vi "Lab Panel V5.40.vi"() -> ()   [LabVIEW 2017] (continued)
                                frame "CHART TEST", Default {
                                }
                                frame "CYCLE TEST" {
                                }
                                frame "T-RISE TEST" {
                                }
                                }
                                n851 = Unbundle(w1495) -> ("DESCRIPTION"=w1494:string)  [unwired: 4 out]
                                n852 = Concatenate Strings(w1490, "\\", w1488, w1486, w1487, w1486) -> (w1497:string)
                                n853 = String To Path(string=w1497) -> (path=w1499:path)
                                n854 = Concatenate Strings(w1497, w1496, w1494, "-", w1493, ".tdms") -> (w1485:string)
                                n855 = Create Folder(path (use dialog)=w1499) -> (error out=w1498:errorcluster)  [unwired: 2 in, 2 out]
                                n856 = global write "Global 1.vi" "LAB03-2 FILE"(w1485) -> ()
                                n857 = call <vilib>:"Clear Errors.vi"("error in (no error)"=w1498) -> ()  [unwired: 5 in, 2 out]
                              }
                              frame #1 {
                                (unwired) FALSE
                                n858 = String To Path(string=w1509) -> (path=w1505:path)
                                n859 = TDMS Open(6:FALSE, 10:T22."create or replace" ("operation (0:open)"), 11:w1505) -> (0:w1504:errorcluster, 3:→"TDMS LAB03-2":refnum<k34>)  [unwired: 4 in]
                              }
                              frame #2 {
                                n860 = local read "SET LAB03-2"() -> (w1515:T5)
                                n861 = local read "TDMS LAB03-2"() -> (w1526:refnum<k34>)
                                n862 = Build Array("Testers Name", "Description", "Set Test Cycles", "T-Rise minutes", "T-Rise Deg C") -> (w1516:string[])
                                n863 = Unbundle(w1515) -> ("NAME"=w1514:string, "DESCRIPTION"=w1513:string, "CYCLES"=w1512:dbl, "T-RISE mins"=w1511:dbl, "T-RISE deg C"=w1510:dbl)
                                n864 = Number To Decimal String(number=w1512) -> (decimal integer string=w1525:string)  [unwired: 1 in]
                                n865 = Number To Decimal String(number=w1511) -> (decimal integer string=w1524:string)  [unwired: 1 in]
                                n866 = Number To Decimal String(number=w1510) -> (decimal integer string=w1523:string)  [unwired: 1 in]
                                n867 = Build Array(w1514, w1513, w1525, w1524, w1523) -> (w1522:string[])
                                n868 = TDMS Set Properties(5:w1522, 7:w1516, 11:w1526) -> ()  [unwired: 3 in, 4 out]
                              }
                              frame #3 {
                                n869 = local read "DISP LAB03-2"() -> (w1531:T4)
                                n870 = Concatenate Strings("LAB03-2  ", w1530) -> (w1532:string)
                                n871 = Two Button Dialog(message=w1532, 1:w1528, 2:w1529) -> (T button?=w1534:bool)
                                n872 = case shown="True" w1534 {
                                tunnel: w1531 -> [w1541 w1542]
                                tunnel: [w1541 w1542] -> w1538
                                tunnel: [w1540 w1543] -> w1537
                                tunnel: [w1539 w1543] -> w1536
                                frame False {
                                n873 = Unbundle(w1541) -> ("CYCLE"=w1540:dbl, "MINS"=w1539:dbl)  [unwired: 1 out]
                                }
                                frame True {
                                w1543 = 0.0
                                }
                                }
                                n874 = Bundle(cluster=w1538, "CYCLE"=w1537, "MINS"=w1536, "STATUS"="RUN") -> (w1527:T4)
                                n875 = local write "DISP LAB03-2"(w1527) -> ()
                              }
                              frame #4 {
                                n876 = local read "TEMP START LAB03-2"() -> (w1546:cluster{"TL":dbl, "TN":dbl})
                                n877 = Bundle(cluster=w1546, "TL"=w1544, "TN"=w1544) -> (w1545:cluster{"TL":dbl, "TN":dbl})
                                n878 = local write "TEMP START LAB03-2"(w1545) -> ()
                              }
                            }
                          }
                        }
                      }
                    }
                  }
                }
              }
              event "RUN LAB04-1": Value Change {
                n879 = event-data() -> ("NewVal"=w1551:bool)  [unwired: 1 in, 5 out]
                n880 = local write "run lab04-1"(w1551) -> ()
                n881 = case shown="True" w1551 {
                  tunnel: w1557 -> [_ w1595]
                  tunnel: w1556 -> [_ w1594]
                  tunnel: w1554 -> [w1559 w1593]
                  tunnel: w1555 -> [_ w1592]
                  tunnel: w1553 -> [_ w1591]
                  tunnel: [w1558 w1590] -> w1552
                  tunnel: w1550 -> [_ w1589]
                  tunnel: w1549 -> [_ w1588]
                  tunnel: w1548 -> [_ w1587]
                  tunnel: w1547 -> [_ w1585]
                  frame False {
                    # "stop test"
                    n882 = stacked-sequence {
                      tunnel: w1559 -> [w1568 _]
                      tunnel: [w1560 _] -> w1558
                      frame #0 {
                        n883 = local read "DISP LAB04-1"() -> (w1567:T4)
                        n884 = Unbundle(w1567) -> ("CYCLE"=w1565:dbl, "MINS"=w1566:dbl)  [unwired: 1 out]
                        n885 = case shown="\"CYCLE TEST\"" w1568 {
                          tunnel: w1566 -> [_ _ w1575]
                          tunnel: w1565 -> [w1573 w1574 _]
                          tunnel: [w1573 w1574 w1575] -> w1564
                          frame "CHART TEST", Default {
                          }
                          frame "CYCLE TEST" {
                          }
                          frame "T-RISE TEST" {
                          }
                        }
                        n886 = local read "TDMS LAB04-1"() -> (w1572:refnum<k34>)
                        n887 = Build Array("STOPPED") -> (w1569:string[])
                        n888 = Build Array(w1564) -> (w1563:dbl[])
                        n889 = TDMS Write(0:w1572, 5:"TEST RESULT", 7:w1569, 9:w1563) -> (4:w1561:refnum<k34>, 15:w1562:errorcluster)  [unwired: 2 in, 2 out]
                        n890 = TDMS Close(8:w1562, 11:w1561) -> (0:w1560:errorcluster)  [unwired: 1 out]
                      }
                      frame #1 {
                        n891 = local read "DISP LAB04-1"() -> (w1579:T4)
                        n892 = stacked-sequence {
                          tunnel: "LAB04-1" -> [w1581 w1583]
                          frame #0 {
                            n893 = call "sub vi - defrag tdms v1.vi"("panel id"=w1581) -> ("error out"=w1580:errorcluster)  [unwired: 10 in]
                            n894 = local write "data file error"(w1580) -> ()
                          }
                          frame #1 {
                            n895 = call "Save data file (stop) v3.vi"("panel id"=w1583) -> ("network file save error"=w1582:errorcluster)  [unwired: 9 in, 1 out]
                            n896 = local write "RESULT LAB04-1"(FALSE) -> ()
                            n897 = local write "data file error"(w1582) -> ()
                          }
                        }
                        n898 = Bundle(cluster=w1579, "STATUS"="STOP") -> (w1577:T4)  [unwired: 2 in]
                        n899 = local write "DISP LAB04-1"(w1577) -> ()
                      }
                    }
                  }
                  frame True {
                    n900 = local read "SIG LAB04-1"() -> (w1586:T2)
                    n901 = stacked-sequence {
                      seq-local: [w1597 _] -> [_ w1601]
                      tunnel: w1595 -> [_ w1611]
                      tunnel: w1594 -> [_ w1610]
                      tunnel: w1593 -> [_ w1609]
                      tunnel: w1592 -> [_ w1608]
                      tunnel: w1591 -> [_ w1607]
                      tunnel: [_ w1606] -> w1590
                      tunnel: w1589 -> [_ w1605]
                      tunnel: w1588 -> [_ w1604]
                      tunnel: w1587 -> [_ w1603]
                      tunnel: w1586 -> [w1596 w1602]
                      tunnel: w1585 -> [_ w1600]
                      frame #0 {
                        n902 = Unbundle(w1596) -> ("AMPS"=w1599:dbl)  [unwired: 4 out]
                        n903 = call "Check For Amps on v1.vi"("ID"="LAB04-1", "amps"=w1599) -> ("amps"=w1597:bool)  [unwired: 9 in]
                      }
                      frame #1 {
                        n904 = case shown="True" w1601 {
                          tunnel: w1611 -> [_ w1624]
                          tunnel: w1610 -> [_ w1623]
                          tunnel: w1609 -> [_ w1622]
                          tunnel: w1608 -> [_ w1621]
                          tunnel: w1607 -> [_ w1620]
                          tunnel: [errorcluster {"status"=FALSE, "code"=0, "source"=""} ("error out") w1619] -> w1606
                          tunnel: w1605 -> [_ w1618]
                          tunnel: w1604 -> [_ w1617]
                          tunnel: w1603 -> [_ w1616]
                          tunnel: w1602 -> [_ w1615]
                          tunnel: w1600 -> [_ w1614]
                          frame False {
                            w1612 = FALSE
                            n905 = local write "RUN LAB04-1"(w1612) -> ()
                            n906 = local write "run lab04-1"(w1612) -> ()
                          }
                          frame True {
                            n907 = stacked-sequence {
                              seq-local: [w1625 _ _ _ _] -> [_ w1649 _ _ _]
                              tunnel: w1624 -> [w1630 _ _ _ _]
                              tunnel: w1623 -> [w1626 _ _ _ _]
                              tunnel: w1622 -> [w1640 _ _ _ _]
                              tunnel: w1621 -> [w1633 _ _ _ _]
                              tunnel: w1620 -> [w1628 _ _ _ _]
                              tunnel: [_ w1644 _ _ _] -> w1619
                              tunnel: w1618 -> [_ _ _ w1670 _]
                              tunnel: w1617 -> [_ _ _ w1669 _]
                              tunnel: w1616 -> [_ _ _ w1668 _]
                              tunnel: w1615 -> [_ _ _ _ _]
                              tunnel: w1614 -> [_ _ _ _ w1684]
                              frame #0 {
                                w1627 = "\\"
                                n908 = local read "SET LAB04-1"() -> (w1635:T5)
                                n909 = case shown="\"CYCLE TEST\"" w1640 {
                                tunnel: ["L04-1-CHART TEST-" "L04-1-CYCLE TEST-" "L04-1-T-RISE TEST-"] -> w1636
                                frame "CHART TEST", Default {
                                }
                                frame "CYCLE TEST" {
                                }
                                frame "T-RISE TEST" {
                                }
                                }
                                n910 = Unbundle(w1635) -> ("DESCRIPTION"=w1634:string)  [unwired: 4 out]
                                n911 = Concatenate Strings(w1630, "\\", w1628, w1627, w1626, w1627) -> (w1637:string)
                                n912 = String To Path(string=w1637) -> (path=w1639:path)
                                n913 = Concatenate Strings(w1637, w1636, w1634, "-", w1633, ".tdms") -> (w1625:string)
                                n914 = Create Folder(path (use dialog)=w1639) -> (error out=w1638:errorcluster)  [unwired: 2 in, 2 out]
                                n915 = global write "Global 1.vi" "LAB04-1 FILE"(w1625) -> ()
                                n916 = call <vilib>:"Clear Errors.vi"("error in (no error)"=w1638) -> ()  [unwired: 5 in, 2 out]
                              }
                              frame #1 {
                                (unwired) FALSE
                                n917 = String To Path(string=w1649) -> (path=w1645:path)
                                n918 = TDMS Open(6:FALSE, 10:T22."create or replace" ("operation (0:open)"), 11:w1645) -> (0:w1644:errorcluster, 3:→"TDMS LAB04-1":refnum<k34>)  [unwired: 4 in]
                              }
                              frame #2 {
                                n919 = local read "SET LAB04-1"() -> (w1655:T5)
                                n920 = local read "TDMS LAB04-1"() -> (w1666:refnum<k34>)
                                n921 = Build Array("Testers Name", "Description", "Set Test Cycles", "T-Rise minutes", "T-Rise Deg C") -> (w1656:string[])
                                n922 = Unbundle(w1655) -> ("NAME"=w1654:string, "DESCRIPTION"=w1653:string, "CYCLES"=w1652:dbl, "T-RISE mins"=w1651:dbl, "T-RISE deg C"=w1650:dbl)
                                n923 = Number To Decimal String(number=w1652) -> (decimal integer string=w1665:string)  [unwired: 1 in]
                                n924 = Number To Decimal String(number=w1651) -> (decimal integer string=w1664:string)  [unwired: 1 in]
                                n925 = Number To Decimal String(number=w1650) -> (decimal integer string=w1663:string)  [unwired: 1 in]
                                n926 = Build Array(w1654, w1653, w1665, w1664, w1663) -> (w1662:string[])
                                n927 = TDMS Set Properties(5:w1662, 7:w1656, 11:w1666) -> ()  [unwired: 3 in, 4 out]
                              }
                              frame #3 {
                                n928 = local read "DISP LAB04-1"() -> (w1671:T4)
                                n929 = Concatenate Strings("LAB04-1  ", w1670) -> (w1672:string)
                                n930 = Two Button Dialog(message=w1672, 1:w1668, 2:w1669) -> (T button?=w1674:bool)
                                n931 = case shown="True" w1674 {
                                tunnel: w1671 -> [w1681 w1682]
                                tunnel: [w1681 w1682] -> w1678
                                tunnel: [w1680 w1683] -> w1677
                                tunnel: [w1679 w1683] -> w1676
                                frame False {
                                n932 = Unbundle(w1681) -> ("CYCLE"=w1680:dbl, "MINS"=w1679:dbl)  [unwired: 1 out]
                                }
                                frame True {
                                w1683 = 0.0
                                }
                                }
                                n933 = Bundle(cluster=w1678, "CYCLE"=w1677, "MINS"=w1676, "STATUS"="RUN") -> (w1667:T4)
                                n934 = local write "DISP LAB04-1"(w1667) -> ()
                              }
                              frame #4 {
                                n935 = local read "TEMP START LAB04-1"() -> (w1686:cluster{"TL":dbl, "TN":dbl})
                                n936 = Bundle(cluster=w1686, "TL"=w1684, "TN"=w1684) -> (w1685:cluster{"TL":dbl, "TN":dbl})
                                n937 = local write "TEMP START LAB04-1"(w1685) -> ()
                              }
                            }
                          }
                        }
                      }
                    }
                  }
                }
              }
              event "RUN LAB04-2": Value Change {
                n938 = event-data() -> ("NewVal"=w1691:bool)  [unwired: 1 in, 5 out]
                n939 = local write "run lab04-2"(w1691) -> ()
                n940 = case shown="True" w1691 {
                  tunnel: w1697 -> [_ w1735]
                  tunnel: w1696 -> [_ w1734]
                  tunnel: w1694 -> [w1699 w1733]
                  tunnel: w1695 -> [_ w1732]
                  tunnel: w1693 -> [_ w1731]
                  tunnel: [w1698 w1730] -> w1692
                  tunnel: w1690 -> [_ w1729]
                  tunnel: w1689 -> [_ w1728]
                  tunnel: w1688 -> [_ w1727]
                  tunnel: w1687 -> [_ w1725]
                  frame False {
                    # "stop test"
                    n941 = stacked-sequence {
                      tunnel: w1699 -> [w1708 _]
                      tunnel: [w1700 _] -> w1698
                      frame #0 {
                        n942 = local read "DISP LAB04-2"() -> (w1707:T4)
                        n943 = Unbundle(w1707) -> ("CYCLE"=w1705:dbl, "MINS"=w1706:dbl)  [unwired: 1 out]
                        n944 = case shown="\"CYCLE TEST\"" w1708 {
                          tunnel: w1706 -> [_ _ w1715]
                          tunnel: w1705 -> [w1713 w1714 _]
                          tunnel: [w1713 w1714 w1715] -> w1704
                          frame "CHART TEST", Default {
                          }
                          frame "CYCLE TEST" {
                          }
                          frame "T-RISE TEST" {
                          }
                        }
                        n945 = local read "TDMS LAB04-2"() -> (w1712:refnum<k34>)
                        n946 = Build Array("STOPPED") -> (w1709:string[])
                        n947 = Build Array(w1704) -> (w1703:dbl[])
                        n948 = TDMS Write(0:w1712, 5:"TEST RESULT", 7:w1709, 9:w1703) -> (4:w1701:refnum<k34>, 15:w1702:errorcluster)  [unwired: 2 in, 2 out]
                        n949 = TDMS Close(8:w1702, 11:w1701) -> (0:w1700:errorcluster)  [unwired: 1 out]
                      }
                      frame #1 {
                        n950 = local read "DISP LAB04-2"() -> (w1719:T4)
                        n951 = stacked-sequence {
                          tunnel: "LAB04-2" -> [w1721 w1723]
                          frame #0 {
                            n952 = call "sub vi - defrag tdms v1.vi"("panel id"=w1721) -> ("error out"=w1720:errorcluster)  [unwired: 10 in]
                            n953 = local write "data file error"(w1720) -> ()
                          }
                          frame #1 {
                            n954 = call "Save data file (stop) v3.vi"("panel id"=w1723) -> ("network file save error"=w1722:errorcluster)  [unwired: 9 in, 1 out]
                            n955 = local write "RESULT LAB04-2"(FALSE) -> ()
                            n956 = local write "data file error"(w1722) -> ()
                          }
                        }
                        n957 = Bundle(cluster=w1719, "STATUS"="STOP") -> (w1717:T4)  [unwired: 2 in]
                        n958 = local write "DISP LAB04-2"(w1717) -> ()
                      }
                    }
                  }
                  frame True {
                    n959 = local read "SIG LAB04-2"() -> (w1726:T2)
                    n960 = stacked-sequence {
                      seq-local: [w1737 _] -> [_ w1741]
                      tunnel: w1735 -> [_ w1751]
                      tunnel: w1734 -> [_ w1750]
                      tunnel: w1733 -> [_ w1749]
                      tunnel: w1732 -> [_ w1748]
                      tunnel: w1731 -> [_ w1747]
                      tunnel: [_ w1746] -> w1730
                      tunnel: w1729 -> [_ w1745]
                      tunnel: w1728 -> [_ w1744]
                      tunnel: w1727 -> [_ w1743]
                      tunnel: w1726 -> [w1736 w1742]
                      tunnel: w1725 -> [_ w1740]
                      frame #0 {
                        n961 = Unbundle(w1736) -> ("AMPS"=w1739:dbl)  [unwired: 4 out]
                        n962 = call "Check For Amps on v1.vi"("ID"="LAB04-2", "amps"=w1739) -> ("amps"=w1737:bool)  [unwired: 9 in]
                      }
                      frame #1 {
                        n963 = case shown="True" w1741 {
                          tunnel: w1751 -> [_ w1764]
                          tunnel: w1750 -> [_ w1763]
                          tunnel: w1749 -> [_ w1762]
                          tunnel: w1748 -> [_ w1761]
                          tunnel: w1747 -> [_ w1760]
                          tunnel: [errorcluster {"status"=FALSE, "code"=0, "source"=""} ("error out") w1759] -> w1746
                          tunnel: w1745 -> [_ w1758]
                          tunnel: w1744 -> [_ w1757]
                          tunnel: w1743 -> [_ w1756]
                          tunnel: w1742 -> [_ w1755]
                          tunnel: w1740 -> [_ w1754]
                          frame False {
                            w1752 = FALSE
                            n964 = local write "RUN LAB04-2"(w1752) -> ()
                            n965 = local write "run lab04-2"(w1752) -> ()
                          }
                          frame True {
                            n966 = stacked-sequence {
                              seq-local: [w1765 _ _ _ _] -> [_ w1789 _ _ _]
                              tunnel: w1764 -> [w1770 _ _ _ _]
                              tunnel: w1763 -> [w1766 _ _ _ _]
                              tunnel: w1762 -> [w1780 _ _ _ _]
                              tunnel: w1761 -> [w1773 _ _ _ _]
                              tunnel: w1760 -> [w1768 _ _ _ _]
                              tunnel: [_ w1784 _ _ _] -> w1759
                              tunnel: w1758 -> [_ _ _ w1810 _]
                              tunnel: w1757 -> [_ _ _ w1809 _]
                              tunnel: w1756 -> [_ _ _ w1808 _]
                              tunnel: w1755 -> [_ _ _ _ _]
                              tunnel: w1754 -> [_ _ _ _ w1824]
                              frame #0 {
                                w1767 = "\\"
                                n967 = local read "SET LAB04-2"() -> (w1775:T5)
                                n968 = case shown="\"CHART TEST\", Default" w1780 {
                                tunnel: ["L04-2-CHART TEST-" "L04-2-CYCLE TEST-" "L04-2-T-RISE TEST-"] -> w1776
                                frame "CHART TEST", Default {
                                }
                                frame "CYCLE TEST" {
                                }
                                frame "T-RISE TEST" {
                                }
                                }
                                n969 = Unbundle(w1775) -> ("DESCRIPTION"=w1774:string)  [unwired: 4 out]
                                n970 = Concatenate Strings(w1770, "\\", w1768, w1767, w1766, w1767) -> (w1777:string)
                                n971 = String To Path(string=w1777) -> (path=w1779:path)
                                n972 = Concatenate Strings(w1777, w1776, w1774, "-", w1773, ".tdms") -> (w1765:string)
                                n973 = Create Folder(path (use dialog)=w1779) -> (error out=w1778:errorcluster)  [unwired: 2 in, 2 out]
                                n974 = global write "Global 1.vi" "LAB04-2 FILE"(w1765) -> ()
                                n975 = call <vilib>:"Clear Errors.vi"("error in (no error)"=w1778) -> ()  [unwired: 5 in, 2 out]
                              }
                              frame #1 {
                                (unwired) FALSE
                                n976 = String To Path(string=w1789) -> (path=w1785:path)
                                n977 = TDMS Open(6:FALSE, 10:T22."create or replace" ("operation (0:open)"), 11:w1785) -> (0:w1784:errorcluster, 3:→"TDMS LAB04-2":refnum<k34>)  [unwired: 4 in]
                              }
                              frame #2 {
                                n978 = local read "SET LAB04-2"() -> (w1795:T5)
                                n979 = local read "TDMS LAB04-2"() -> (w1806:refnum<k34>)
                                n980 = Build Array("Testers Name", "Description", "Set Test Cycles", "T-Rise minutes", "T-Rise Deg C") -> (w1796:string[])
                                n981 = Unbundle(w1795) -> ("NAME"=w1794:string, "DESCRIPTION"=w1793:string, "CYCLES"=w1792:dbl, "T-RISE mins"=w1791:dbl, "T-RISE deg C"=w1790:dbl)
                                n982 = Number To Decimal String(number=w1792) -> (decimal integer string=w1805:string)  [unwired: 1 in]
                                n983 = Number To Decimal String(number=w1791) -> (decimal integer string=w1804:string)  [unwired: 1 in]
                                n984 = Number To Decimal String(number=w1790) -> (decimal integer string=w1803:string)  [unwired: 1 in]
                                n985 = Build Array(w1794, w1793, w1805, w1804, w1803) -> (w1802:string[])
                                n986 = TDMS Set Properties(5:w1802, 7:w1796, 11:w1806) -> ()  [unwired: 3 in, 4 out]
                              }
                              frame #3 {
                                n987 = local read "DISP LAB04-2"() -> (w1811:T4)
                                n988 = Concatenate Strings("LAB04-2 ", w1810) -> (w1812:string)
                                n989 = Two Button Dialog(message=w1812, 1:w1808, 2:w1809) -> (T button?=w1814:bool)
                                n990 = case shown="True" w1814 {
                                tunnel: w1811 -> [w1821 w1822]
                                tunnel: [w1821 w1822] -> w1818
                                tunnel: [w1820 w1823] -> w1817
                                tunnel: [w1819 w1823] -> w1816
                                frame False {
                                n991 = Unbundle(w1821) -> ("CYCLE"=w1820:dbl, "MINS"=w1819:dbl)  [unwired: 1 out]
                                }
                                frame True {
                                w1823 = 0.0
                                }
                                }
                                n992 = Bundle(cluster=w1818, "CYCLE"=w1817, "MINS"=w1816, "STATUS"="RUN") -> (w1807:T4)
                                n993 = local write "DISP LAB04-2"(w1807) -> ()
                              }
                              frame #4 {
                                n994 = local read "TEMP START LAB04-2"() -> (w1826:cluster{"TL":dbl, "TN":dbl})
                                n995 = Bundle(cluster=w1826, "TL"=w1824, "TN"=w1824) -> (w1825:cluster{"TL":dbl, "TN":dbl})
                                n996 = local write "TEMP START LAB04-2"(w1825) -> ()
                              }
                            }
                          }
                        }
                      }
                    }
                  }
                }
              }
              event "RUN LAB05-1": Value Change {
                n997 = event-data() -> ("NewVal"=w1831:bool)  [unwired: 1 in, 5 out]
                n998 = local write "run lab05-1"(w1831) -> ()
                n999 = case shown="True" w1831 {
                  tunnel: w1837 -> [_ w1875]
                  tunnel: w1836 -> [_ w1874]
                  tunnel: w1834 -> [w1839 w1873]
                  tunnel: w1835 -> [_ w1872]
                  tunnel: w1833 -> [_ w1871]
                  tunnel: [w1838 w1870] -> w1832
                  tunnel: w1830 -> [_ w1869]
                  tunnel: w1829 -> [_ w1868]
                  tunnel: w1828 -> [_ w1867]
                  tunnel: w1827 -> [_ w1865]
                  frame False {
                    # "stop test"
                    n1000 = stacked-sequence {
                      tunnel: w1839 -> [w1848 _]
                      tunnel: [w1840 _] -> w1838
                      frame #0 {
                        n1001 = local read "DISP LAB05-1"() -> (w1847:T4)
                        n1002 = Unbundle(w1847) -> ("CYCLE"=w1845:dbl, "MINS"=w1846:dbl)  [unwired: 1 out]
                        n1003 = case shown="\"CYCLE TEST\"" w1848 {
                          tunnel: w1846 -> [_ _ w1855]
                          tunnel: w1845 -> [w1853 w1854 _]
                          tunnel: [w1853 w1854 w1855] -> w1844
                          frame "CHART TEST", Default {
                          }
                          frame "CYCLE TEST" {
                          }
                          frame "T-RISE TEST" {
                          }
                        }
                        n1004 = local read "TDMS LAB05-1"() -> (w1852:refnum<k34>)
                        n1005 = Build Array("STOPPED") -> (w1849:string[])
                        n1006 = Build Array(w1844) -> (w1843:dbl[])
                        n1007 = TDMS Write(0:w1852, 5:"TEST RESULT", 7:w1849, 9:w1843) -> (4:w1841:refnum<k34>, 15:w1842:errorcluster)  [unwired: 2 in, 2 out]
                        n1008 = TDMS Close(8:w1842, 11:w1841) -> (0:w1840:errorcluster)  [unwired: 1 out]
                      }
                      frame #1 {
                        n1009 = local read "DISP LAB05-1"() -> (w1859:T4)
                        n1010 = stacked-sequence {
                          tunnel: "LAB05-1" -> [w1861 w1863]
                          frame #0 {
                            n1011 = call "sub vi - defrag tdms v1.vi"("panel id"=w1861) -> ("error out"=w1860:errorcluster)  [unwired: 10 in]
                            n1012 = local write "data file error"(w1860) -> ()
                          }
                          frame #1 {
                            n1013 = call "Save data file (stop) v3.vi"("panel id"=w1863) -> ("network file save error"=w1862:errorcluster)  [unwired: 9 in, 1 out]
                            n1014 = local write "RESULT LAB05-1"(FALSE) -> ()
                            n1015 = local write "data file error"(w1862) -> ()
                          }
                        }
                        n1016 = Bundle(cluster=w1859, "STATUS"="STOP") -> (w1857:T4)  [unwired: 2 in]
                        n1017 = local write "DISP LAB05-1"(w1857) -> ()
                      }
                    }
                  }
                  frame True {
                    n1018 = local read "SIG LAB05-1"() -> (w1866:T2)
                    n1019 = stacked-sequence {
                      seq-local: [w1877 _] -> [_ w1881]
                      tunnel: w1875 -> [_ w1891]
                      tunnel: w1874 -> [_ w1890]
                      tunnel: w1873 -> [_ w1889]
                      tunnel: w1872 -> [_ w1888]
                      tunnel: w1871 -> [_ w1887]
                      tunnel: [_ w1886] -> w1870
                      tunnel: w1869 -> [_ w1885]
                      tunnel: w1868 -> [_ w1884]
                      tunnel: w1867 -> [_ w1883]
                      tunnel: w1866 -> [w1876 w1882]
                      tunnel: w1865 -> [_ w1880]
                      frame #0 {
                        n1020 = Unbundle(w1876) -> ("AMPS"=w1879:dbl)  [unwired: 4 out]
                        n1021 = call "Check For Amps on v1.vi"("ID"="LAB05-1", "amps"=w1879) -> ("amps"=w1877:bool)  [unwired: 9 in]
                      }
                      frame #1 {
                        n1022 = case shown="True" w1881 {
                          tunnel: w1891 -> [_ w1904]
                          tunnel: w1890 -> [_ w1903]
                          tunnel: w1889 -> [_ w1902]
                          tunnel: w1888 -> [_ w1901]
                          tunnel: w1887 -> [_ w1900]
                          tunnel: [errorcluster {"status"=FALSE, "code"=0, "source"=""} ("error out") w1899] -> w1886
                          tunnel: w1885 -> [_ w1898]
                          tunnel: w1884 -> [_ w1897]
                          tunnel: w1883 -> [_ w1896]
                          tunnel: w1882 -> [_ w1895]
                          tunnel: w1880 -> [_ w1894]
                          frame False {
                            w1892 = FALSE
                            n1023 = local write "RUN LAB05-1"(w1892) -> ()
                            n1024 = local write "run lab05-1"(w1892) -> ()
                          }
                          frame True {
                            n1025 = stacked-sequence {
                              seq-local: [w1905 _ _ _ _] -> [_ w1929 _ _ _]
                              tunnel: w1904 -> [w1910 _ _ _ _]
                              tunnel: w1903 -> [w1906 _ _ _ _]
                              tunnel: w1902 -> [w1920 _ _ _ _]
                              tunnel: w1901 -> [w1913 _ _ _ _]
                              tunnel: w1900 -> [w1908 _ _ _ _]
                              tunnel: [_ w1924 _ _ _] -> w1899
                              tunnel: w1898 -> [_ _ _ w1949 _]
                              tunnel: w1897 -> [_ _ _ w1948 _]
                              tunnel: w1896 -> [_ _ _ w1947 _]
                              tunnel: w1895 -> [_ _ _ _ _]
                              tunnel: w1894 -> [_ _ _ _ w1964]
                              frame #0 {
                                w1907 = "\\"
                                n1026 = local read "SET LAB05-1"() -> (w1915:T5)
                                n1027 = case shown="\"CYCLE TEST\"" w1920 {
                                tunnel: ["L05-1-CHART TEST-" "L05-1-CYCLE TEST-" "L05-1-T-RISE TEST-"] -> w1916
                                frame "CHART TEST", Default {
                                }
                                frame "CYCLE TEST" {
                                }
                                frame "T-RISE TEST" {
                                }
                                }
                                n1028 = Unbundle(w1915) -> ("DESCRIPTION"=w1914:string)  [unwired: 4 out]
                                n1029 = Concatenate Strings(w1910, "\\", w1908, w1907, w1906, w1907) -> (w1917:string)
                                n1030 = String To Path(string=w1917) -> (path=w1919:path)
                                n1031 = Concatenate Strings(w1917, w1916, w1914, "-", w1913, ".tdms") -> (w1905:string)
                                n1032 = Create Folder(path (use dialog)=w1919) -> (error out=w1918:errorcluster)  [unwired: 2 in, 2 out]
                                n1033 = global write "Global 1.vi" "LAB05-1 FILE"(w1905) -> ()
                                n1034 = call <vilib>:"Clear Errors.vi"("error in (no error)"=w1918) -> ()  [unwired: 5 in, 2 out]
                              }
                              frame #1 {
                                (unwired) FALSE
                                n1035 = String To Path(string=w1929) -> (path=w1925:path)
                                n1036 = TDMS Open(6:FALSE, 10:T22."create or replace" ("operation (0:open)"), 11:w1925) -> (0:w1924:errorcluster, 3:→"TDMS LAB05-1":refnum<k34>)  [unwired: 4 in]
                              }
                              frame #2 {
                                n1037 = local read "SET LAB05-1"() -> (w1935:T5)
                                n1038 = local read "TDMS LAB05-1"() -> (w1946:refnum<k34>)
                                n1039 = Build Array("Testers Name", "Description", "Set Test Cycles", "T-Rise minutes", "T-Rise Deg C") -> (w1936:string[])
                                n1040 = Unbundle(w1935) -> ("NAME"=w1934:string, "DESCRIPTION"=w1933:string, "CYCLES"=w1932:dbl, "T-RISE mins"=w1931:dbl, "T-RISE deg C"=w1930:dbl)
                                n1041 = Number To Decimal String(number=w1932) -> (decimal integer string=w1945:string)  [unwired: 1 in]
                                n1042 = Number To Decimal String(number=w1931) -> (decimal integer string=w1944:string)  [unwired: 1 in]
                                n1043 = Number To Decimal String(number=w1930) -> (decimal integer string=w1943:string)  [unwired: 1 in]
                                n1044 = Build Array(w1934, w1933, w1945, w1944, w1943) -> (w1942:string[])
                                n1045 = TDMS Set Properties(5:w1942, 7:w1936, 11:w1946) -> ()  [unwired: 3 in, 4 out]
                              }
                              frame #3 {
                                n1046 = local read "DISP LAB05-1"() -> (w1951:T4)
                                n1047 = Concatenate Strings("LAB05-1  ", w1949) -> (w1952:string)
                                n1048 = Two Button Dialog(message=w1952, 1:w1947, 2:w1948) -> (T button?=w1954:bool)
                                n1049 = case shown="True" w1954 {
                                tunnel: w1951 -> [w1961 w1962]
                                tunnel: [w1961 w1962] -> w1958
                                tunnel: [w1960 w1963] -> w1957
                                tunnel: [w1959 w1963] -> w1956
                                frame False {
                                n1050 = Unbundle(w1961) -> ("CYCLE"=w1960:dbl, "MINS"=w1959:dbl)  [unwired: 1 out]
                                }
                                frame True {
                                w1963 = 0.0
                                }
                                }
                                n1051 = Bundle(cluster=w1958, "CYCLE"=w1957, "MINS"=w1956, "STATUS"="RUN") -> (w1950:T4)
                                n1052 = local write "DISP LAB05-1"(w1950) -> ()
                              }
                              frame #4 {
                                n1053 = local read "TEMP START LAB05-1"() -> (w1966:cluster{"TL":dbl, "TN":dbl})
                                n1054 = Bundle(cluster=w1966, "TL"=w1964, "TN"=w1964) -> (w1965:cluster{"TL":dbl, "TN":dbl})
                                n1055 = local write "TEMP START LAB05-1"(w1965) -> ()
                              }
                            }
                          }
                        }
                      }
                    }
                  }
                }
              }
              event "RUN LAB05-2": Value Change {
                n1056 = event-data() -> ("NewVal"=w1972:bool)  [unwired: 1 in, 5 out]
                n1057 = local read "SIG LAB05-2"() -> (w1968:T2)
                n1058 = case shown="True" w1972 {
                  tunnel: w1978 -> [_ w2016]
                  tunnel: w1977 -> [_ w2015]
                  tunnel: w1975 -> [w1980 w2014]
                  tunnel: w1976 -> [_ w2013]
                  tunnel: w1974 -> [_ w2012]
                  tunnel: [w1979 w2011] -> w1973
                  tunnel: w1971 -> [_ w2010]
                  tunnel: w1970 -> [_ w2009]
                  tunnel: w1969 -> [_ w2008]
                  tunnel: w1968 -> [_ w2007]
                  tunnel: w1967 -> [_ w2006]
                  frame False {
                    # "stop test"
                    n1059 = stacked-sequence {
                      tunnel: w1980 -> [w1989 _]
                      tunnel: [w1981 _] -> w1979
                      frame #0 {
                        n1060 = local read "DISP LAB05-2"() -> (w1988:T4)
                        n1061 = Unbundle(w1988) -> ("CYCLE"=w1986:dbl, "MINS"=w1987:dbl)  [unwired: 1 out]
                        n1062 = case shown="\"CYCLE TEST\"" w1989 {
                          tunnel: w1987 -> [_ _ w1996]
                          tunnel: w1986 -> [w1994 w1995 _]
                          tunnel: [w1994 w1995 w1996] -> w1985
                          frame "CHART TEST", Default {
                          }
                          frame "CYCLE TEST" {
                          }
                          frame "T-RISE TEST" {
                          }
                        }
                        n1063 = local read "TDMS LAB05-2"() -> (w1993:refnum<k34>)
                        n1064 = Build Array("STOPPED") -> (w1990:string[])
                        n1065 = Build Array(w1985) -> (w1984:dbl[])
                        n1066 = TDMS Write(0:w1993, 5:"TEST RESULT", 7:w1990, 9:w1984) -> (4:w1982:refnum<k34>, 15:w1983:errorcluster)  [unwired: 2 in, 2 out]
                        n1067 = TDMS Close(8:w1983, 11:w1982) -> (0:w1981:errorcluster)  [unwired: 1 out]
                      }
                      frame #1 {
                        n1068 = local read "DISP LAB05-2"() -> (w2000:T4)
                        n1069 = stacked-sequence {
                          tunnel: "LAB05-2" -> [w2002 w2004]
                          frame #0 {
                            n1070 = call "sub vi - defrag tdms v1.vi"("panel id"=w2002) -> ("error out"=w2001:errorcluster)  [unwired: 10 in]
                            n1071 = local write "data file error"(w2001) -> ()
                          }
                          frame #1 {
                            n1072 = local write "RESULT LAB05-2"(FALSE) -> ()
                            n1073 = call "Save data file (stop) v3.vi"("panel id"=w2004) -> ("network file save error"=w2003:errorcluster)  [unwired: 9 in, 1 out]
                            n1074 = local write "data file error"(w2003) -> ()
                          }
                        }
                        n1075 = Bundle(cluster=w2000, "STATUS"="STOP") -> (w1998:T4)  [unwired: 2 in]
                        n1076 = local write "DISP LAB05-2"(w1998) -> ()
                      }
                    }
                  }
                  frame True {
                    n1077 = stacked-sequence {
                      seq-local: [w2018 _] -> [_ w2022]
                      tunnel: w2016 -> [_ w2032]
                      tunnel: w2015 -> [_ w2031]
                      tunnel: w2014 -> [_ w2030]
                      tunnel: w2013 -> [_ w2029]
                      tunnel: w2012 -> [_ w2028]
                      tunnel: [_ w2027] -> w2011
                      tunnel: w2010 -> [_ w2026]
                      tunnel: w2009 -> [_ w2025]
                      tunnel: w2008 -> [_ w2024]
                      tunnel: w2007 -> [w2017 w2023]
                      tunnel: w2006 -> [_ w2021]
                      frame #0 {
                        n1078 = Unbundle(w2017) -> ("AMPS"=w2020:dbl)  [unwired: 4 out]
                        n1079 = call "Check For Amps on v1.vi"("ID"="LAB05-2", "amps"=w2020) -> ("amps"=w2018:bool)  [unwired: 9 in]
                      }
                      frame #1 {
                        n1080 = case shown="True" w2022 {
                          tunnel: w2032 -> [_ w2044]
                          tunnel: w2031 -> [_ w2042]
                          tunnel: w2030 -> [_ w2039]
                          tunnel: w2029 -> [_ w2040]
                          tunnel: w2028 -> [_ w2043]
                          tunnel: [errorcluster {"status"=FALSE, "code"=0, "source"=""} ("error out") w2035] -> w2027
                          tunnel: w2026 -> [_ w2038]
                          tunnel: w2025 -> [_ w2037]
                          tunnel: w2024 -> [_ w2036]
                          tunnel: w2023 -> [_ w2041]
                          tunnel: w2021 -> [_ w2045]
                          frame False {
                            w2033 = FALSE
                            n1081 = local write "RUN LAB05-2"(w2033) -> ()
                            n1082 = local write "run lab05-2"(w2033) -> ()
                          }
                          frame True {
                            n1083 = stacked-sequence {
                              seq-local: [w2046 _ _ _ _] -> [_ w2070 _ _ _]
                              tunnel: w2044 -> [w2051 _ _ _ _]
                              tunnel: w2042 -> [w2047 _ _ _ _]
                              tunnel: w2039 -> [w2061 _ _ _ _]
                              tunnel: w2040 -> [w2054 _ _ _ _]
                              tunnel: w2043 -> [w2049 _ _ _ _]
                              tunnel: [_ w2065 _ _ _] -> w2035
                              tunnel: w2038 -> [_ _ _ w2090 _]
                              tunnel: w2037 -> [_ _ _ w2089 _]
                              tunnel: w2036 -> [_ _ _ w2088 _]
                              tunnel: w2041 -> [_ _ _ _ _]
                              tunnel: w2045 -> [_ _ _ _ w2105]
                              frame #0 {
                                w2048 = "\\"
                                n1084 = local read "SET LAB05-2"() -> (w2056:T5)
                                n1085 = case shown="\"CYCLE TEST\"" w2061 {
                                tunnel: ["L05-2-CHART TEST-" "L05-2-CYCLE TEST-" "L05-2-T-RISE TEST-"] -> w2057
                                frame "CHART TEST", Default {
                                }
                                frame "CYCLE TEST" {
                                }
                                frame "T-RISE TEST" {
                                }
                                }
                                n1086 = Unbundle(w2056) -> ("DESCRIPTION"=w2055:string)  [unwired: 4 out]
                                n1087 = Concatenate Strings(w2051, "\\", w2049, w2048, w2047, w2048) -> (w2058:string)
                                n1088 = String To Path(string=w2058) -> (path=w2060:path)
                                n1089 = Concatenate Strings(w2058, w2057, w2055, "-", w2054, ".tdms") -> (w2046:string)
                                n1090 = Create Folder(path (use dialog)=w2060) -> (error out=w2059:errorcluster)  [unwired: 2 in, 2 out]
                                n1091 = global write "Global 1.vi" "LAB05-2 FILE"(w2046) -> ()
                                n1092 = call <vilib>:"Clear Errors.vi"("error in (no error)"=w2059) -> ()  [unwired: 5 in, 2 out]
                              }
                              frame #1 {
                                (unwired) FALSE
                                n1093 = String To Path(string=w2070) -> (path=w2066:path)
                                n1094 = TDMS Open(6:FALSE, 10:T22."create or replace" ("operation (0:open)"), 11:w2066) -> (0:w2065:errorcluster, 3:→"TDMS LAB05-2":refnum<k34>)  [unwired: 4 in]
                              }
                              frame #2 {
                                n1095 = local read "SET LAB05-2"() -> (w2076:T5)
                                n1096 = local read "TDMS LAB05-2"() -> (w2087:refnum<k34>)
                                n1097 = Build Array("Testers Name", "Description", "Set Test Cycles", "T-Rise minutes", "T-Rise Deg C") -> (w2077:string[])
                                n1098 = Unbundle(w2076) -> ("NAME"=w2075:string, "DESCRIPTION"=w2074:string, "CYCLES"=w2073:dbl, "T-RISE mins"=w2072:dbl, "T-RISE deg C"=w2071:dbl)
                                n1099 = Number To Decimal String(number=w2073) -> (decimal integer string=w2086:string)  [unwired: 1 in]
                                n1100 = Number To Decimal String(number=w2072) -> (decimal integer string=w2085:string)  [unwired: 1 in]
                                n1101 = Number To Decimal String(number=w2071) -> (decimal integer string=w2084:string)  [unwired: 1 in]
                                n1102 = Build Array(w2075, w2074, w2086, w2085, w2084) -> (w2083:string[])
                                n1103 = TDMS Set Properties(5:w2083, 7:w2077, 11:w2087) -> ()  [unwired: 3 in, 4 out]
                              }
                              frame #3 {
                                n1104 = local read "DISP LAB05-2"() -> (w2092:T4)
                                n1105 = Concatenate Strings("LAB05-2  ", w2090) -> (w2093:string)
                                n1106 = Two Button Dialog(message=w2093, 1:w2088, 2:w2089) -> (T button?=w2095:bool)
                                n1107 = case shown="True" w2095 {
                                tunnel: w2092 -> [w2102 w2103]
                                tunnel: [w2102 w2103] -> w2099
                                tunnel: [w2101 w2104] -> w2098
                                tunnel: [w2100 w2104] -> w2097
                                frame False {
                                n1108 = Unbundle(w2102) -> ("CYCLE"=w2101:dbl, "MINS"=w2100:dbl)  [unwired: 1 out]
                                }
                                frame True {
                                w2104 = 0.0
                                }
                                }
                                n1109 = Bundle(cluster=w2099, "CYCLE"=w2098, "MINS"=w2097, "STATUS"="RUN") -> (w2091:T4)
                                n1110 = local write "DISP LAB05-2"(w2091) -> ()
                              }
                              frame #4 {
                                n1111 = local read "TEMP START LAB05-2"() -> (w2107:cluster{"TL":dbl, "TN":dbl})
                                n1112 = Bundle(cluster=w2107, "TL"=w2105, "TN"=w2105) -> (w2106:cluster{"TL":dbl, "TN":dbl})
                                n1113 = local write "TEMP START LAB05-2"(w2106) -> ()
                              }
                            }
                          }
                        }
                      }
                    }
                  }
                }
                n1114 = local write "run lab05-2"(w1972) -> ()
              }
            }
            n1115 = local write "data file error"(w676) -> ()
          }
          frame #5 {
            # "Check if test cycles reached for cycle tests, if so then test pass"
            n1116 = stacked-sequence {
              tunnel: w2127 -> [_ _ _ _ _ _ _ _ _ _]
              tunnel: w2126 -> [_ _ _ _ _ _ _ _ _ _]
              tunnel: w2125 -> [_ _ _ _ _ _ _ _ _ _]
              tunnel: w2124 -> [_ _ _ _ _ _ _ _ _ _]
              tunnel: w2123 -> [_ _ _ _ _ _ _ _ _ _]
              tunnel: w2122 -> [_ _ _ _ _ _ _ _ _ _]
              tunnel: w2121 -> [_ _ _ _ _ _ _ _ _ _]
              tunnel: w2120 -> [_ _ _ _ _ _ _ _ _ _]
              tunnel: w2119 -> [_ _ _ _ _ _ _ _ _ _]
              tunnel: w2118 -> [_ _ _ _ _ _ _ _ _ _]
              tunnel: w2117 -> [w2133 _ _ _ _ _ _ _ _ _]
              tunnel: w2116 -> [_ w2168 _ _ _ _ _ _ _ _]
              tunnel: w2115 -> [_ _ w2208 _ _ _ _ _ _ _]
              tunnel: w2114 -> [_ _ _ w2248 _ _ _ _ _ _]
              tunnel: w2113 -> [_ _ _ _ w2288 _ _ _ _ _]
              tunnel: w2112 -> [_ _ _ _ _ w2328 _ _ _ _]
              tunnel: w2111 -> [_ _ _ _ _ _ w2368 _ _ _]
              tunnel: w2110 -> [_ _ _ _ _ _ _ w2408 _ _]
              tunnel: w2109 -> [_ _ _ _ _ _ _ _ w2448 _]
              tunnel: w2108 -> [_ _ _ _ _ _ _ _ _ w2488]
              frame #0 {
                # "LAB01-1"
                n1117 = Less?(x=w2133, y=2) -> (x < y?=w2131:bool)
                n1118 = local read "DISP LAB01-1"() -> (w2134:T4)
                n1119 = Unbundle By Name(w2134) -> ("STATUS"=w2128:string)
